vi "Start Logger.vi"(8 "error in (no error)":errorcluster, 11 "Pulse Controller in":refnum<class "Pulse Controller.lvclass">) -> (0 "error out":errorcluster, 3 "Pulse Controller out":refnum<class "Pulse Controller.lvclass">)   [LabVIEW 2015, in "Pulse Controller.lvclass"]
uses:
  Pulse Controller.lvclass
  Measure Object/Measure Object.lvclass/Measure Object.ctl
  Measure Object/Write tdms stream.vi
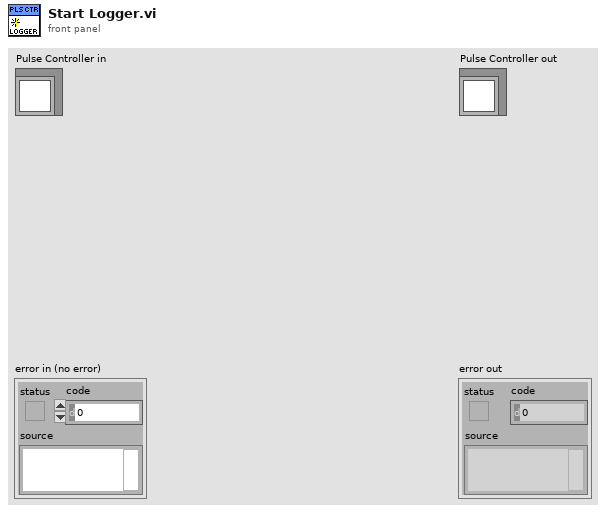
[diagram p1: front panel]
types:
  T1 = enum16{"open", "open or create", "create or replace", "create", "open (read-only)"}
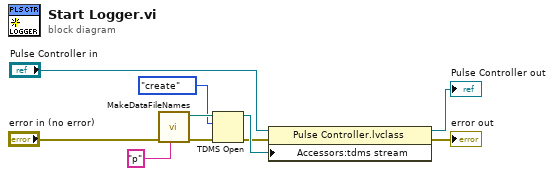
[diagram p0: block diagram]
diagram:
  n1 = call "MakeDataFileNames.vi"("File Prefix"="p", "Error In"="error in (no error)") -> ("Error Out"=w7:errorcluster, "Data File  Path"=w9:path)  [unwired: 6 in, 2 out]
  n2 = TDMS Open(8:w7, 10:T1."create" ("operation (0:open)"), 11:w9) -> (0:w3:errorcluster, 3:w4:refnum<k34>)  [unwired: 4 in]
  n3 = property class="Pulse Controller.lvclass"(reference="Pulse Controller in", error in=w3, "Accessors:tdms stream"=w4) -> (reference out=→"Pulse Controller out":refnum<class "Pulse Controller.lvclass">, error out=→"error out":errorcluster)
